vi "set distance type.vi"(0 "index_id":u64, 3 "Overwrite Lib Path":path, 5 "distance type":T1=1 items=["EUCLIDEAN"=1, "MANHATTAN"=2, "MINKOWSKY"=3, "HIST INTERSECT"=5, "HELLINGER"=6, "CHI SQUARE"=7, "KULLBACK LEIBLER"=8], 7 "Minkowsky Order":i32, 11 "error in (no error)":errorcluster) -> (4 "index_id out":u64, 15 "error out":errorcluster)   [LabVIEW 2020, in "KD Tree.lvlib"]
uses:
  KD Tree.lvlib
  Distance Type.ctl
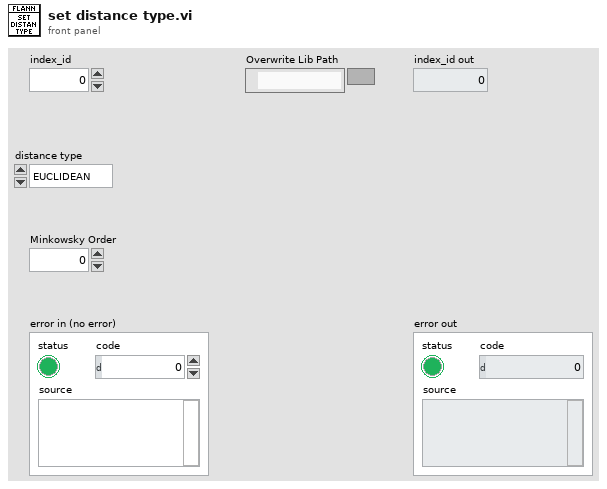
[diagram p1: front panel]
types:
  T1 = typedef "KD Tree.lvlib/Distance Type.ctl" = u32
  T2 = typedef "Semaphore RefNum" = refnum<k1>
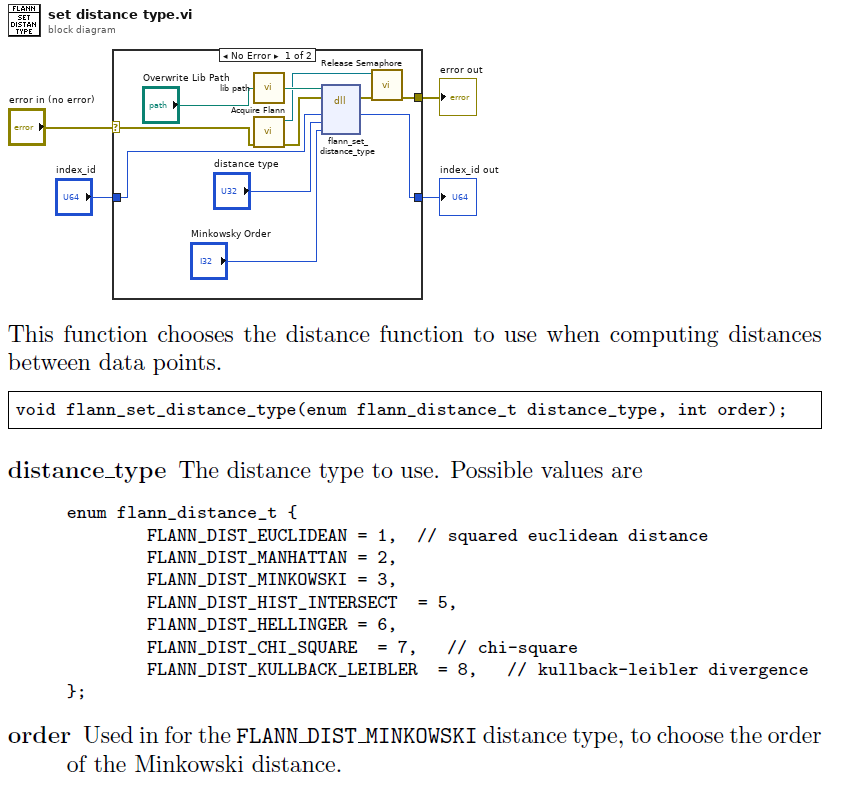
[diagram p0: block diagram]
diagram:
  n1 = case shown="No Error" "error in (no error)" {
    selector: "error in (no error)" -> [w14 w17]
    tunnel: [w15 w16] -> w4
    tunnel: [w6 w17] -> w2
    tunnel: "index_id" -> [w12 w16]
    frame No Error {
      n2 = call "lib path.vi"("Overwrite Lib Path"="Overwrite Lib Path") -> ("lib path"=w11:path)
      n3 = call "Acquire Flann.vi"("error in (no error)"=w14) -> ("error out"=w7:errorcluster, "semaphore"=w5:T2)  [unwired: 9 in]
      n4 = dll-call lib="E:/Labview/LV 2020/Libs/flann/flann.dll" fn="flann_set_distance_type"(path in=w11, error in=w7, "index_id"=w12, "distance_type"="distance type", "order"="Minkowsky Order") -> (error out=w13:errorcluster, "index_id"=w15:u64)  [unwired: 4 in, 1 out]
      n5 = call <vilib>:"Release Semaphore.vi"("error in (no error)"=w13, "semaphore"=w5) -> ("error out"=w6:errorcluster)  [unwired: 4 in, 1 out]
    }
    frame Error {
    }
  }
  "index_id out" <- w4
  "error out" <- w2
